vi "get_dcMeasurement.vi"(0 "NInstrSim_ReadDCMeasurement":refnum<class "NInstrSim_ReadDCMeasurement.lvclass">, 5 "error in (no error)":errorcluster) -> (14 "dup NInstrSim_ReadDCMeasurement":refnum<class "NInstrSim_ReadDCMeasurement.lvclass">, 16 "dcMeasurement":dbl format="%_6g", 19 "error out":errorcluster)   [LabVIEW 2009, in "HB_Device_Examples.lvlib" / "NInstrSim_ReadDCMeasurement.lvclass"]
doc: "This VI retruns the result of the DC Measurement."
uses:
  NInstrSim_ReadDCMeasurement.lvclass
  NInstrSim_ReadDCMeasurement.lvclass/NInstrSim_ReadDCMeasurement.ctl
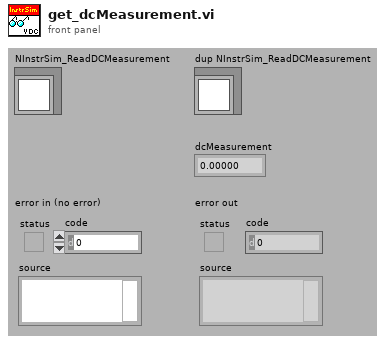
[diagram p1: front panel]
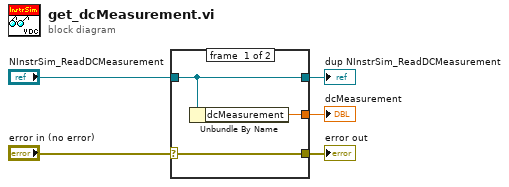
[diagram p0: block diagram]
diagram:
  n1 = case shown="No Error" "error in (no error)" {
    selector: "error in (no error)" -> [w8 w9]
    tunnel: [w8 w9] -> w4
    tunnel: [w7 w10] -> w2
    tunnel: "NInstrSim_ReadDCMeasurement" -> [w7 w10]
    tunnel: [w6 _] -> w1
    frame #0 {
      n2 = Unbundle By Name(w7) -> ("dcMeasurement"=w6:dbl)
    }
    frame #1 {
    }
  }
  "error out" <- w4
  "dup NInstrSim_ReadDCMeasurement" <- w2
  "dcMeasurement" <- w1
